vi "draw -- set cursors for lorenzian.vi"(7 "action":enum16{"gamma omega", "4corners", "a"}(ring)=enum."a", 9 "lorentzian":T1={"A (VHz)"=-1.0311345636926572, "f (Hz)"=-1.0311345636926572, "G (Hz)"=-1.0311345636926572, "phi(rad)"=-1.0311345636926572, "Q"=-1.0311345636926572, "Norm  Ampl"=-1.0311345636926572, "bg (V)"=-1.0311345636926572+0.0i, "4corners"={"z (-pi/2)"=-1.0311345636926572+0.5736824521422934i, "z(inf)"=-0.5200164984937075+1.0975277942502903i, "z (pi/2)"=-1.0311345636926572+0.5736824521422934i, "z center"=-0.5136528600391839+0.580046090596817i, "z(0)"=-0.5200164984937075+1.0975277942502903i, "radius"=-1.0311345636926572}} {"bg (V)" format="%#9_9f"; "Q" format="%#9_9f"; "phi(rad)" format="%#9_9f"; "G (Hz)" format="%#9_9f"; "f (Hz)" format="%#9_9f"}, 11 "Plot":refnum<vi>) -> ()   [LabVIEW 2018]
uses:
  circle corners.ctl
  lorentzian.ctl
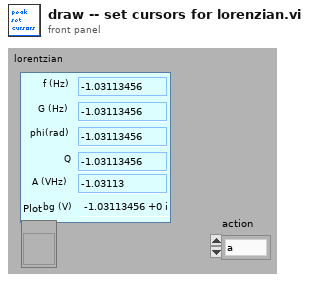
[diagram p1: front panel]
types:
  T1 = typedef "lorentzian.ctl" = cluster{"A (VHz)":dbl, "f (Hz)":dbl, "G (Hz)":dbl, "phi(rad)":dbl, "Q":dbl, "Norm  Ampl":dbl, "bg (V)":cdb, "4corners":T2}
  T2 = typedef "circle corners.ctl" = cluster{"z (-pi/2)":cdb, "z(inf)":cdb, "z (pi/2)":cdb, "z center":cdb, "z(0)":cdb, "radius":dbl}
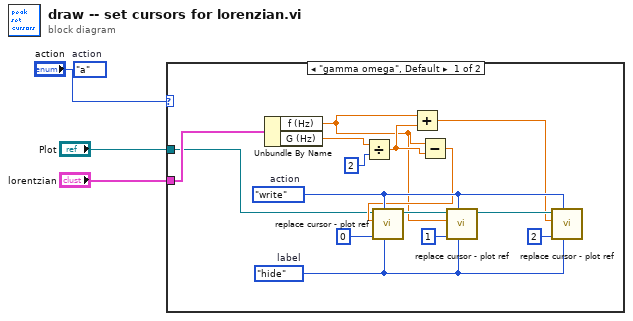
[diagram p0: block diagram]
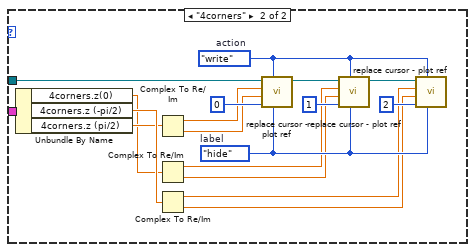
[diagram p2: hidden frame]
diagram:
  (unwired) enum16{"gamma omega", "4corners", "a"}."a"  # action
  n1 = case shown="\"gamma omega\", Default" "action" {
    tunnel: "Plot" -> [w4 w29]
    tunnel: "lorentzian" -> [w5 w20]
    frame "gamma omega", Default {
      w12 = enum16{"hide", "show x", "show y", "show (x,y)"}."hide"  # label
      w18 = enum16{"", "read", "write"}."write"  # action
      n2 = Unbundle By Name(w5) -> ("f (Hz)"=w7:dbl, "G (Hz)"=w6:dbl)
      n3 = Divide(x=w6, y=2) -> (x/y=w10:dbl)
      n4 = Add(x=w7, y=w10) -> (x+y=w9:dbl)
      n5 = Subtract(x=w7, y=w10) -> (x-y=w8:dbl)
      n6 = call "replace cursor - plot ref.vi"("label"=w12, "action"=w18, "cursor index"=0, "new X"=w8, "Plot ref in"=w4) -> ("Plot ref out"=w14:refnum<vi>)  [unwired: 4 in, 2 out]
      n7 = call "replace cursor - plot ref.vi"("label"=w12, "action"=w18, "cursor index"=1, "new X"=w7, "Plot ref in"=w14) -> ("Plot ref out"=w13:refnum<vi>)  [unwired: 4 in, 2 out]
      n8 = call "replace cursor - plot ref.vi"("label"=w12, "action"=w18, "cursor index"=2, "new X"=w9, "Plot ref in"=w13) -> ()  [unwired: 4 in, 3 out]
    }
    frame "4corners" {
      w30 = enum16{"hide", "show x", "show y", "show (x,y)"}."hide"  # label
      w36 = enum16{"", "read", "write"}."write"  # action
      n9 = Unbundle By Name(w20) -> ("4corners.z(0)"=w19:cdb, "4corners.z (-pi/2)"=w22:cdb, "4corners.z (pi/2)"=w21:cdb)
      n10 = Complex To Re/Im(x + iy=w21) -> (x=w28:dbl, y=w27:dbl)
      n11 = Complex To Re/Im(x + iy=w19) -> (x=w26:dbl, y=w25:dbl)
      n12 = Complex To Re/Im(x + iy=w22) -> (x=w24:dbl, y=w23:dbl)
      n13 = call "replace cursor - plot ref.vi"("label"=w30, "action"=w36, "cursor index"=0, "new  Y"=w27, "new X"=w28, "Plot ref in"=w29) -> ("Plot ref out"=w32:refnum<vi>)  [unwired: 3 in, 2 out]
      n14 = call "replace cursor - plot ref.vi"("label"=w30, "action"=w36, "cursor index"=1, "new  Y"=w25, "new X"=w26, "Plot ref in"=w32) -> ("Plot ref out"=w31:refnum<vi>)  [unwired: 3 in, 2 out]
      n15 = call "replace cursor - plot ref.vi"("label"=w30, "action"=w36, "cursor index"=2, "new  Y"=w23, "new X"=w24, "Plot ref in"=w31) -> ()  [unwired: 3 in, 3 out]
    }
  }
